vi "FL Set Variable.vi"(0 "fuzzy system in":T4 {"user MF interpolating polynomials"."coa_x(y) coeff" format="%.4g"; "user MF interpolating polynomials"."Area(y) coeff" format="%.4g"; "user MF interpolating polynomials"."X(y) coeff" format="%.4g"; "user MF interpolating polynomials"."Y(x) coeff" format="%.4g"; "user MF interpolating polynomials"."Y" format="%.4g"; "user MF interpolating polynomials"."X" format="%.4g"; "defuzzification method" items=["Center of Area", "Modified Center of Area", "Center of Sums", "Center of Maximum", "Mean of Maximum"]; "rules"."consequents"."Var Index" min=0; "rules"."consequents"."Cond" items=["=", "!="]; "rules"."consequents"."MF Index" min=0; "rules"."antecedents"."Var Index" min=0; "rules"."antecedents"."Cond" items=["=", "!="]; "rules"."antecedents"."MF Index" min=0; "rules"."consequent implication" items=["Minimum", "Product"]; "rules"."antecedent connective" items=["AND (Minimum)", "AND (Product)", "OR (Maximum)", "OR (Probabilistic)"]; "output variables"."MFs"."shape" items=["Triangle", "Trapezoid", "Singleton", "Sigmoid", "Gaussian", "User-Defined"]; "input variables"."MFs"."shape" items=["Triangle", "Trapezoid", "Singleton", "Sigmoid", "Gaussian", "User-Defined"]}, 1 "input/output":T1 items=["Input", "Output"], 2 "variable index":i32, 5 "name":string, 7 "minimum":dbl, 9 "maximum":dbl, 11 "error in (no error)":errorcluster, 12 "membership functions":T2[](array[typedef])=[{"name"="<>", "shape"=0, "points"=[], "color"=16448250, "user-defined shape index"=0}] {"shape" items=["Triangle", "Trapezoid", "Singleton", "Sigmoid", "Gaussian", "User-Defined"]}) -> (4 "fuzzy system out":T4 {"user MF interpolating polynomials"."coa_x(y) coeff" format="%.4g"; "user MF interpolating polynomials"."Area(y) coeff" format="%.4g"; "user MF interpolating polynomials"."X(y) coeff" format="%.4g"; "user MF interpolating polynomials"."Y(x) coeff" format="%.4g"; "user MF interpolating polynomials"."Y" format="%.4g"; "user MF interpolating polynomials"."X" format="%.4g"; "defuzzification method" items=["Center of Area", "Modified Center of Area", "Center of Sums", "Center of Maximum", "Mean of Maximum"]; "rules"."consequents"."Var Index" min=0; "rules"."consequents"."Cond" items=["=", "!="]; "rules"."consequents"."MF Index" min=0; "rules"."antecedents"."Var Index" min=0; "rules"."antecedents"."Cond" items=["=", "!="]; "rules"."antecedents"."MF Index" min=0; "rules"."consequent implication" items=["Minimum", "Product"]; "rules"."antecedent connective" items=["AND (Minimum)", "AND (Product)", "OR (Maximum)", "OR (Probabilistic)"]; "output variables"."MFs"."shape" items=["Triangle", "Trapezoid", "Singleton", "Sigmoid", "Gaussian", "User-Defined"]; "input variables"."MFs"."shape" items=["Triangle", "Trapezoid", "Singleton", "Sigmoid", "Gaussian", "User-Defined"]}, 15 "error out":errorcluster)   [LabVIEW 2017, in "NI_Fuzzy_Logic_API.lvlib"]
doc: "Modifies the name, range, or membership functions of a linguistic variable in a fuzzy system."
uses:
  <vilib>/addons/Fuzzy Logic/NI_Fuzzy_Logic_API.lvlib
  <vilib>/addons/Fuzzy Logic/TypeDefs/FL System.ctl
  <vilib>/addons/Fuzzy Logic/TypeDefs/FL Variable.ctl
  <vilib>/addons/Fuzzy Logic/TypeDefs/FL Membership Function.ctl
  <vilib>/addons/Fuzzy Logic/TypeDefs/FL Membership Function Shape.ctl
  <vilib>/addons/Fuzzy Logic/TypeDefs/FL Rule.ctl
  <vilib>/addons/Fuzzy Logic/TypeDefs/FL Antecedent.ctl
  <vilib>/addons/Fuzzy Logic/TypeDefs/FL Modifier.ctl
  <vilib>/addons/Fuzzy Logic/TypeDefs/FL Antecedent Connective.ctl
  <vilib>/addons/Fuzzy Logic/TypeDefs/FL Consequent.ctl
  <vilib>/addons/Fuzzy Logic/TypeDefs/FL Consequent Implication.ctl
  <vilib>/addons/Fuzzy Logic/TypeDefs/FL Defuzzification.ctl
  <vilib>/addons/Fuzzy Logic/TypeDefs/FL Interpolating polynomials.ctl
  <vilib>/addons/Fuzzy Logic/TypeDefs/FL Input_Output.ctl
panel:
  # "A single memberhip function with the name <> and empty points array is the default value of this control and indicates that nothing was connected to it, then the memberhip functions array will not be edited."
  # "IF"
  # "THEN"
  # "IF"
  # "THEN"
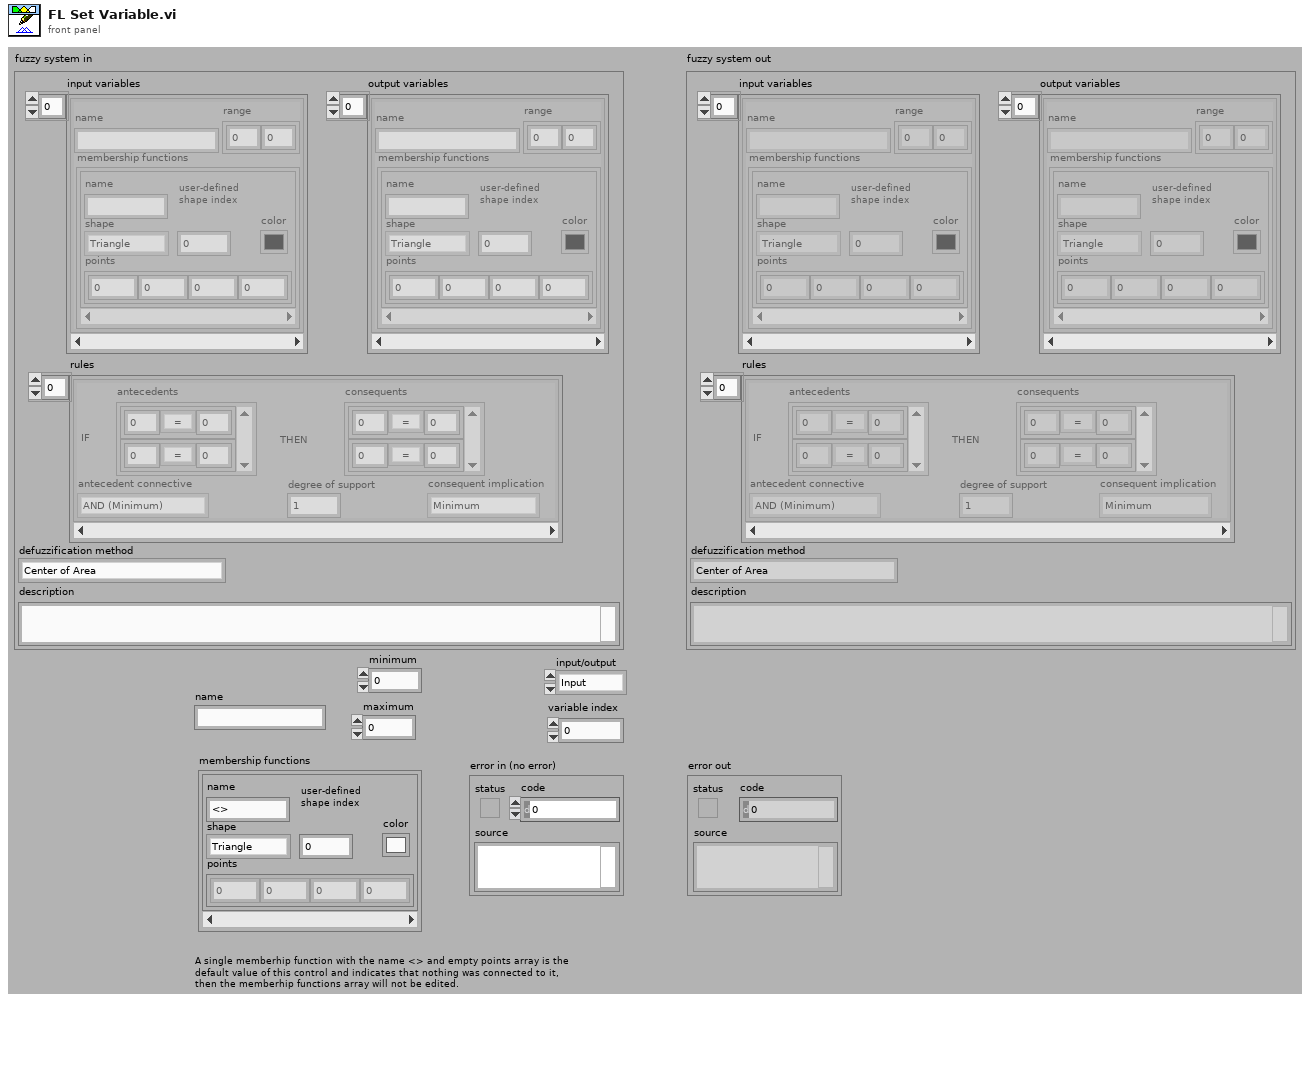
[diagram p1: front panel]
types:
  T1 = typedef "NI_Fuzzy_Logic_API.lvlib/FL Input_Output.ctl" = u16
  T2 = typedef "NI_Fuzzy_Logic_API.lvlib/FL Membership Function.ctl" = cluster{"name":string, "shape":T3, "points":dbl[], "color":u32, "user-defined shape index":i32}
  T3 = typedef "NI_Fuzzy_Logic_API.lvlib/FL Membership Function Shape.ctl" = u16
  T4 = typedef "NI_Fuzzy_Logic_API.lvlib/FL System.ctl" = cluster{"input variables":T5[], "output variables":T5[], "rules":T6[], "defuzzification method":T12, "description":string, "user MF interpolating polynomials":T13[]}
  T5 = typedef "NI_Fuzzy_Logic_API.lvlib/FL Variable.ctl" = cluster{"name":string, "range":dbl[], "MFs":T2[]}
  T6 = typedef "NI_Fuzzy_Logic_API.lvlib/FL Rule.ctl" = cluster{"antecedents":T7[], "antecedent connective":T9, "consequents":T10[], "consequent implication":T11, "degree of support":dbl}
  T7 = typedef "NI_Fuzzy_Logic_API.lvlib/FL Antecedent.ctl" = cluster{"Var Index":i32, "MF Index":i32, "Cond":T8}
  T8 = typedef "NI_Fuzzy_Logic_API.lvlib/FL Modifier.ctl" = u16
  T9 = typedef "NI_Fuzzy_Logic_API.lvlib/FL Antecedent Connective.ctl" = u16
  T10 = typedef "NI_Fuzzy_Logic_API.lvlib/FL Consequent.ctl" = cluster{"Var Index":i32, "MF Index":i32, "Cond":T8}
  T11 = typedef "NI_Fuzzy_Logic_API.lvlib/FL Consequent Implication.ctl" = u16
  T12 = typedef "NI_Fuzzy_Logic_API.lvlib/FL Defuzzification.ctl" = u16
  T13 = typedef "NI_Fuzzy_Logic_API.lvlib/FL Interpolating polynomials.ctl" = cluster{"X":dbl[], "Y":dbl[], "Y(x) coeff":dbl[][], "X(y) coeff":dbl[][], "Area(y) coeff":dbl[][], "coa_x(y) coeff":dbl[][]}
  T14 = cluster{"name":string, "range":dbl[], "membership functions":T2[]}
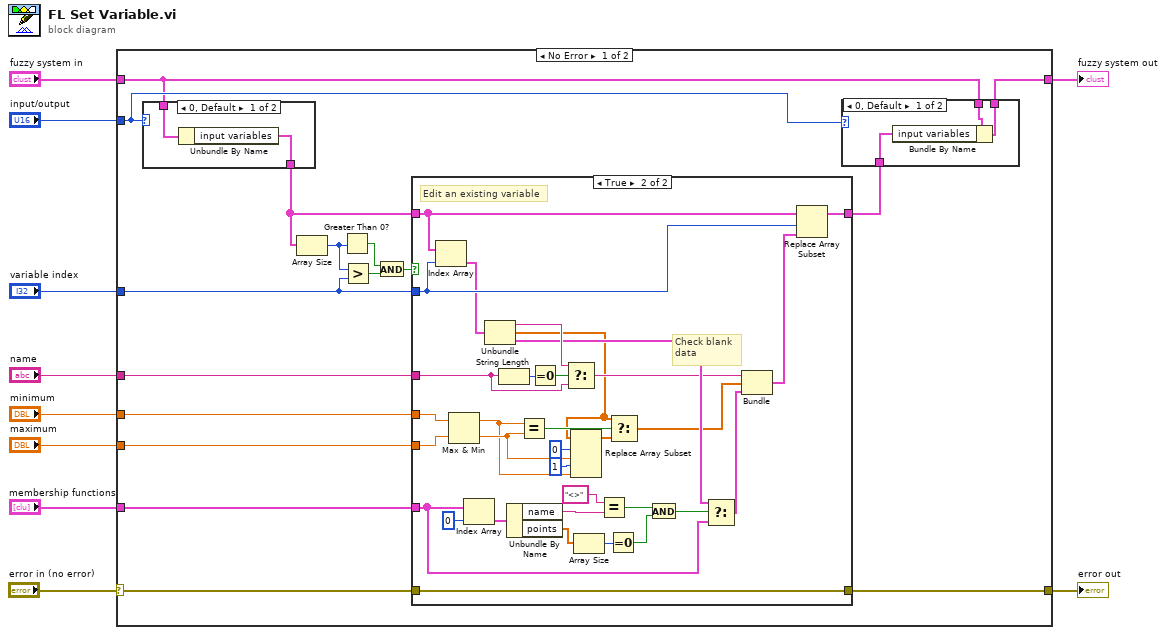
[diagram p0: block diagram]
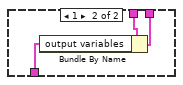
[diagram p2: hidden frame]
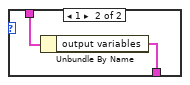
[diagram p3: hidden frame]
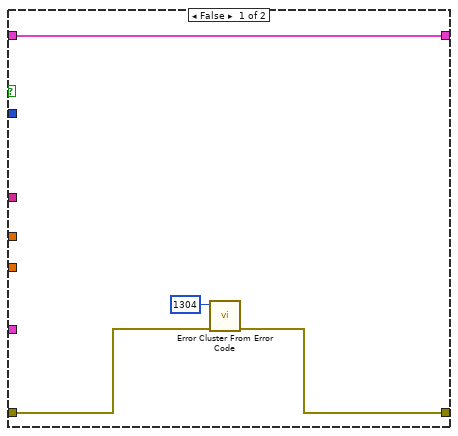
[diagram p4: hidden frame]
diagram:
  n1 = case shown="No Error" "error in (no error)" {
    selector: "error in (no error)" -> [w14 w75]
    tunnel: "variable index" -> [w22 _]
    tunnel: "name" -> [w16 _]
    tunnel: "membership functions" -> [w15 _]
    tunnel: "input/output" -> [w19 _]
    tunnel: [w18 w74] -> w6
    tunnel: "fuzzy system in" -> [w17 w74]
    tunnel: [w13 w75] -> w3
    tunnel: "minimum" -> [w12 _]
    tunnel: "maximum" -> [w11 _]
    frame No Error {
      n2 = case shown="0, Default" w19 {
        tunnel: [w34 w35] -> w21
        tunnel: w17 -> [w33 w36]
        frame 0, Default {
          n3 = Unbundle By Name(w33) -> ("input variables"=w34:T5[])
        }
        frame 1 {
          n4 = Unbundle By Name(w36) -> ("output variables"=w35:T5[])
        }
      }
      n5 = Array Size(array=w21) -> (size(s)=w25:i32)
      n6 = Greater Than 0?(x=w25) -> (x > 0?=w24:bool)
      n7 = Greater?(x=w25, y=w22) -> (0:w26:bool)
      n8 = And(x=w24, y=w26) -> (x .and. y?=w23:bool)
      n9 = case shown="True" w23 {
        tunnel: w22 -> [_ w71]
        tunnel: [w40 w73] -> w20
        tunnel: w21 -> [w40 w72]
        tunnel: w16 -> [_ w65]
        tunnel: w15 -> [_ w50]
        tunnel: w14 -> [w39 w60]
        tunnel: [w38 w60] -> w13
        tunnel: w12 -> [_ w55]
        tunnel: w11 -> [_ w54]
        frame False {
          n10 = call <vilib>:"Error Cluster From Error Code.vi"("error in (no error)"=w39, "error code (0)"=1304) -> ("error out"=w38:errorcluster)  [unwired: 1 in, 6 out]
        }
        frame True {
          # "Check blank\ndata"
          # "Edit an existing variable"
          n11 = Index Array(array=w72, index=w71) -> (element=w68:T5)
          n12 = Max & Min(x=w55, y=w54) -> (max(x,y)=w52:dbl, min(x,y)=w53:dbl)
          n13 = Index Array(array=w50, index=0) -> (element=w48:T2)
          n14 = Unbundle(w68) -> ("name"=w67:string, "range"=w58:dbl[], "MFs"=w66:T2[])
          n15 = String Length(string=w65) -> (length=w70:i32)
          n16 = Unbundle By Name(w48) -> ("name"=w47:string, "points"=w45:dbl[])
          n17 = Equal?(x=w52, y=w53) -> (x = y?=w59:bool)
          n18 = Equal To 0?(x=w70) -> (x = 0?=w69:bool)
          n19 = Select(t=w67, s=w69, f=w65) -> (s? t:f=w64:string)
          n20 = Replace Array Subset(array=w58, new element #1=w53, index #1=0 ("index"), new element #2=w52, index #2=1 ("index")) -> (w51:dbl[])
          n21 = Array Size(array=w45) -> (size(s)=w44:i32)
          n22 = Equal?(x="<>" ("y"), y=w47) -> (x = y?=w43:bool)
          n23 = Equal To 0?(x=w44) -> (x = 0?=w42:bool)
          n24 = Select(t=w58, s=w59, f=w51) -> (s? t:f=w63:dbl[])
          n25 = And(x=w43, y=w42) -> (x .and. y?=w41:bool)
          n26 = Select(t=w66, s=w41, f=w50) -> (s? t:f=w62:T2[])
          n27 = Bundle("name"=w64, "range"=w63, "membership functions"=w62) -> (w61:T14)  [unwired: 1 out]
          n28 = Replace Array Subset(array=w72, new element=w61, index=w71) -> (w73:T5[])
        }
      }
      n29 = case shown="0, Default" w19 {
        tunnel: w20 -> [w29 w32]
        tunnel: [w28 w31] -> w18
        tunnel: w17 -> [w27 w30]
        frame 0, Default {
          n30 = Bundle By Name(cluster=w27, "input variables"=w29) -> (w28:T4)
        }
        frame 1 {
          n31 = Bundle By Name(cluster=w30, "output variables"=w32) -> (w31:T4)
        }
      }
    }
    frame Error {
    }
  }
  "fuzzy system out" <- w6
  "error out" <- w3
